vi "ReadWait.vi"(6 "Numeric":dbl, 8 "error in (no error)":errorcluster, 9 "Value":bool=TRUE, 10 "Read":i32, 11 "I-O in":refnum<class "I-O.lvclass">) -> (0 "error out":errorcluster, 3 "I-O out":refnum<class "I-O.lvclass">)   [LabVIEW 2021, in "I-O.lvclass"]
uses:
  I-O.lvclass
  <vilib>/Utility/file.llb/Read Delimited Spreadsheet (string).vi
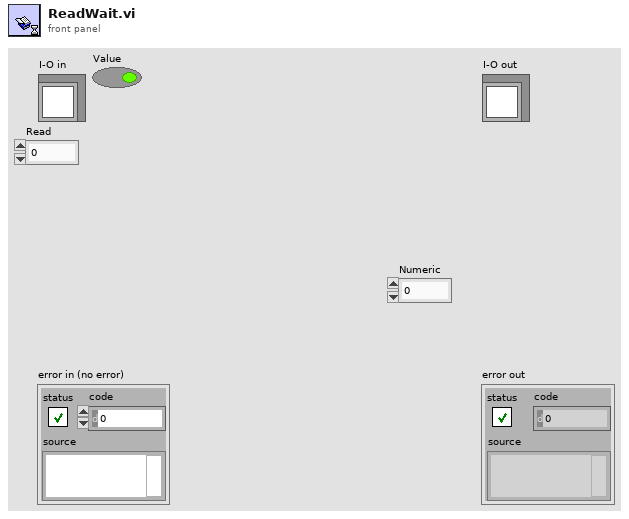
[diagram p1: front panel]
types:
  T1 = typedef "File Paths.ctl" = cluster{"Glue Pattern Folder":path, "Carrier Tray Folder":path, "Pick Up Tool Fixture Folder":path, "Components Folder":path, "Bellows Tool Offset.txt":path, "Pick Up Tool Offset.txt":path, "Dispense Tip Offset.txt":path, "Log Files":path, "Gantry Assembly Map.txt":path, "Syringe and offset map.txt":path, "Controllers Folder":path, "Local dbase config":path}
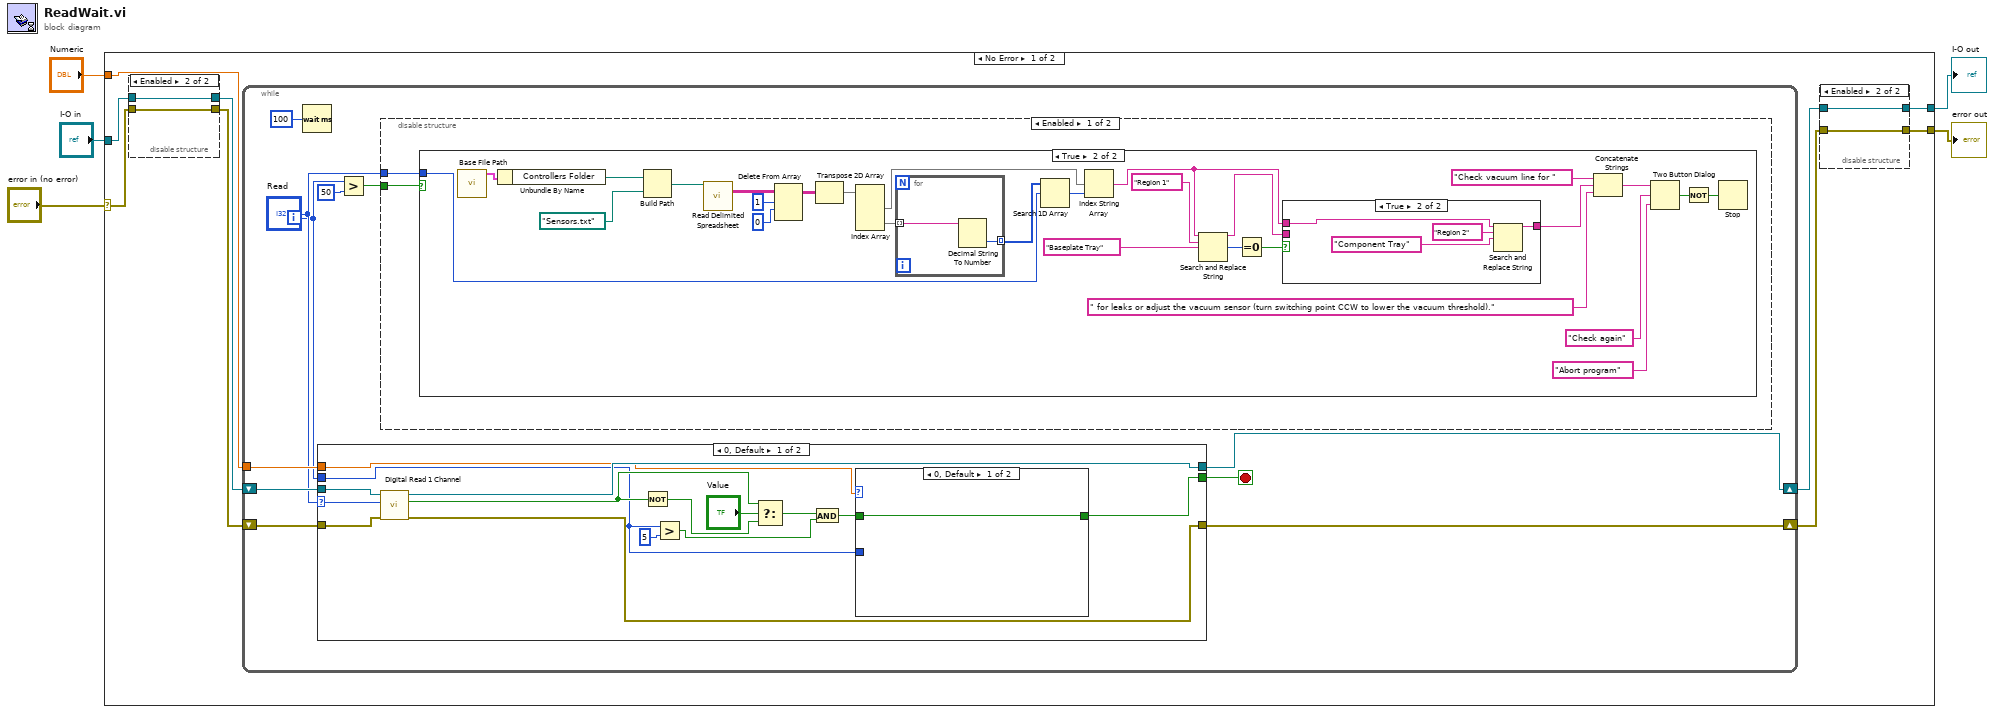
[diagram p0: block diagram]
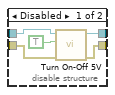
[diagram p2: hidden frame]
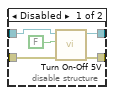
[diagram p3: hidden frame]
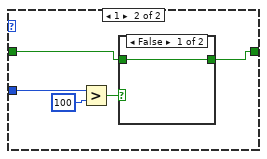
[diagram p7: hidden frame]
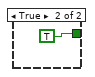
[diagram p8: hidden frame]
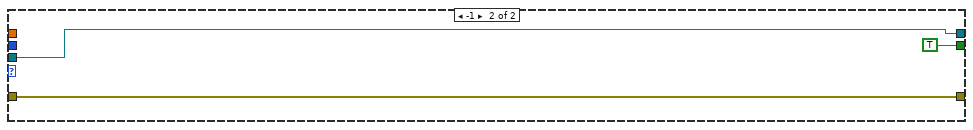
[diagram p9: hidden frame]
diagram:
  n1 = case shown="No Error" "error in (no error)" {
    selector: "error in (no error)" -> [w10 w104]
    tunnel: [w7 w104] -> w4
    tunnel: [w13 w103] -> w2
    tunnel: "I-O in" -> [w14 w103]
    tunnel: "Numeric" -> [w6 _]
    frame No Error {
      n2 = disable-structure shown="Enabled" {
        disable-tunnel: w14 -> [w19 w21]
        disable-tunnel: [w18 w21] -> w12
        disable-tunnel: w10 -> [w17 w20]
        disable-tunnel: [w16 w20] -> w9
        frame Disabled {
          n3 = call-dynamic "Turn On-Off 5V.vi"("error in (no error)"=w17, "Value"=TRUE, "I-O in"=w19) -> ("error out"=w16:errorcluster, "I-O out"=w18:refnum<class "I-O.lvclass">)  [unwired: 7 in]
        }
        frame Enabled {
        }
      }
      n4 = while {
        shift-right: [w37] -> w11
        shift-left: w12 -> [w33]
        shift-right: [w35] -> w8
        shift-left: w9 -> [w36]
        tunnel: w6 -> [w34]
        i -> [w31]
        stop <- w38 stop-if-true
        n5 = Wait (ms)(milliseconds to wait=u32 100) -> ()  [unwired: 1 out]
        n6 = case shown="0, Default" "Read" {
          selector: "Read" -> [w83 _]
          tunnel: w31 -> [w77 _]
          tunnel: [w80 TRUE] -> w38
          tunnel: w33 -> [w87 w102]
          tunnel: [w86 w102] -> w37
          tunnel: w36 -> [w85 w100]
          tunnel: [w84 w100] -> w35
          tunnel: w34 -> [w78 _]
          frame 0, Default {
            n7 = call-dynamic "Digital Read 1 Channel.vi"("error in (no error)"=w85, "Read"=w83, "I-O in"=w87) -> ("error out"=w84:errorcluster, "Value"=w81:bool, "I-O out"=w86:refnum<class "I-O.lvclass">)  [unwired: 6 in]
            n8 = Not(x=w81) -> (.not. x?=w91:bool)
            n9 = Greater?(x=w77, y=5) -> (0:w88:bool)
            n10 = Select(t=w81, s="Value", f=w91) -> (s? t:f=w89:bool)
            n11 = And(x=w89, y=w88) -> (x .and. y?=w79:bool)
            n12 = case shown="0, Default" w78 {
              tunnel: [w92 w97] -> w80
              tunnel: w79 -> [w92 w96]
              tunnel: w77 -> [_ w95]
              frame 0, Default {
              }
              frame 1 {
                n13 = Greater?(x=w95, y=100) -> (0:w94:bool)
                n14 = case shown="False" w94 {
                  tunnel: [w98 TRUE] -> w97
                  tunnel: w96 -> [w98 _]
                  frame False {
                  }
                  frame True {
                  }
                }
              }
            }
          }
          frame -1 {
          }
        }
        n15 = Greater?(x=w31, y=50) -> (0:w29:bool)
        n16 = disable-structure shown="Enabled" {
          disable-tunnel: "Read" -> [w41 _]
          disable-tunnel: w29 -> [w40 _]
          frame Enabled {
            n17 = case shown="True" w40 {
              tunnel: w41 -> [_ w69]
              frame False {
              }
              frame True {
                n18 = call "Base File Path.vi"() -> ("Paths Out"=w68:T1)  [unwired: 11 in]
                n19 = Unbundle By Name(w68) -> ("Controllers Folder"=w67:path)
                n20 = Build Path(base path=w67, name or relative path=path "Sensors.txt") -> (appended path=w65:path)
                n21 = call-poly <vilib>:"Read Delimited Spreadsheet.vi"("file path (dialog if empty)"=w65) -> ("all rows"=w64:string[][])  [unwired: 9 in, 5 out]
                n22 = Delete From Array(array=w64, length=1, index (row)=0) -> (array with subset deleted=w61:string[][])  [unwired: 1 in, 1 out]
                n23 = Transpose 2D Array(2D array=w61) -> (transposed array=w60:string[][])
                n24 = Index Array(array=w60) -> (element #1=w57:string[], element #2=w59:string[])  [unwired: 4 in]
                n25 = for {
                  tunnel: w59 -> [w76] mode=indexing
                  tunnel: [w75] -> w58 mode=indexing
                  n26 = Decimal String To Number(string=w76) -> (number=w75:i32)  [unwired: 2 in, 1 out]
                }
                n27 = Search 1D Array(1D array=w58, element=w69) -> (index of element=w56:i32)  [unwired: 1 in]
                n28 = Index String Array(1:w56, 2:w57) -> (0:w48:string)  [unwired: 1 in]
                n29 = Search and Replace String(input string=w48, search string="Region 1" ("replace string (\"\")"), replace string="Baseplate Tray" ("replace string (\"\")")) -> (result string=w46:string, number of replacements=w50:i32)  [unwired: 5 in, 2 out]
                n30 = Equal To 0?(x=w50) -> (x = 0?=w49:bool)
                n31 = case shown="True" w49 {
                  tunnel: w48 -> [_ w74]
                  tunnel: [w70 w71] -> w47
                  tunnel: w46 -> [w70 _]
                  frame False {
                  }
                  frame True {
                    n32 = Search and Replace String(input string=w74, search string="Region 2", replace string="Component Tray" ("replace string (\"\")")) -> (result string=w71:string)  [unwired: 5 in, 3 out]
                  }
                }
                n33 = Concatenate Strings("Check vacuum line for " ("message"), w47, " for leaks or adjust the vacuum sensor (turn switching point CCW to lower the vacuum threshold)." ("string")) -> (w53:string)
                n34 = Two Button Dialog(message=w53, 1:"Abort program" ("F button name (\"Cancel\")"), 2:"Check again" ("T button name (\"OK\")")) -> (T button?=w43:bool)
                n35 = Not(x=w43) -> (.not. x?=w42:bool)
                n36 = Stop(stop? (T)=w42) -> ()
              }
            }
          }
          frame Disabled {
          }
        }
      }
      n37 = disable-structure shown="Enabled" {
        disable-tunnel: [w26 w28] -> w13
        disable-tunnel: w11 -> [w25 w28]
        disable-tunnel: w8 -> [w24 w27]
        disable-tunnel: [w23 w27] -> w7
        frame Disabled {
          n38 = call-dynamic "Turn On-Off 5V.vi"("error in (no error)"=w24, "Value"=FALSE, "I-O in"=w25) -> ("error out"=w23:errorcluster, "I-O out"=w26:refnum<class "I-O.lvclass">)  [unwired: 7 in]
        }
        frame Enabled {
        }
      }
    }
    frame Error {
    }
  }
  "error out" <- w4
  "I-O out" <- w2
